vi "TimeDelay.vi"(0 "Ground level BP-filter width, Hz":dbl format="%#_13g", 2 "Generator frequency":dbl format="%#_13g", 3 "Sampling frequency":dbl format="%#_13g") -> (1 "dt":dbl format="%#_13g")   [LabVIEW 2015]
uses:
  <vilib>/measure/maspectr.llb/FFT Spectrum (Mag-Phase) for 1 Chan.vi
  <vilib>/Analysis/3filter.llb/Butterworth Filter (DBL).vi
  <vilib>/measure/NI_MABase.lvlib
  <vilib>/measure/NI_MAPro.lvlib
  <vilib>/Analysis/NI_AALBase.lvlib
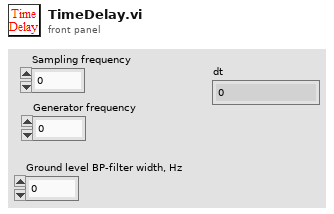
[diagram p1: front panel]
types:
  T1 = cluster{"Sampling frequency":dbl, "Number of samples":dbl}
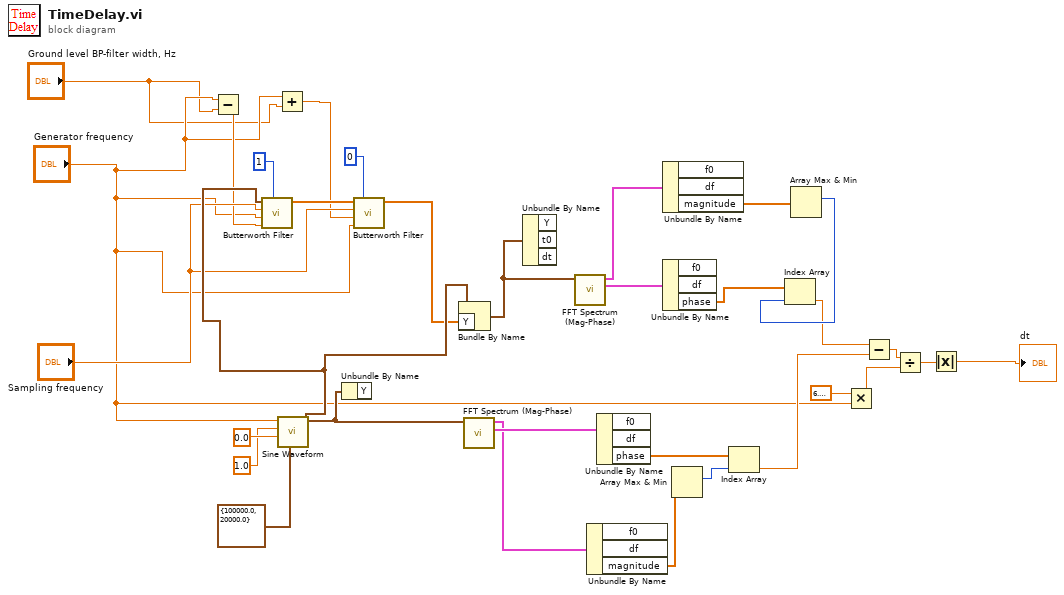
[diagram p0: block diagram]
diagram:
  n1 = Subtract(x="Generator frequency", y="Ground level BP-filter width, Hz") -> (x-y=w5:dbl)
  n2 = Add(x="Generator frequency", y="Ground level BP-filter width, Hz") -> (x+y=w2:dbl)
  n3 = call <vilib>:"Sine Waveform.vi"("sampling info"=T1 {"Sampling frequency"=100000.0, "Number of samples"=20000.0} ("Cluster 2"), "phase"=0.0, "amplitude"=1.0, "frequency"="Generator frequency") -> ("signal out"=w8:waveform(dbl))  [unwired: 6 in, 1 out]
  n4 = call-poly <vilib>:"Butterworth Filter.vi"("filter type"=1, "low cutoff freq: fl"=w5, "high cutoff freq: fh"="Generator frequency", "sampling freq: fs"="Sampling frequency", "X"=w8) -> ("Filtered X"=w11:dbl[])  [unwired: 3 in, 1 out]
  n5 = Unbundle By Name(w8) -> ()  [unwired: 1 out]
  n6 = call-poly <vilib>:"Butterworth Filter.vi"("filter type"=0, "low cutoff freq: fl"="Generator frequency", "high cutoff freq: fh"=w2, "sampling freq: fs"="Sampling frequency", "X"=w11) -> ("Filtered X"=w7:dbl[])  [unwired: 3 in, 1 out]
  n7 = Bundle By Name(cluster=w8, "Y"=w7) -> (w13:waveform(dbl))
  n8 = call-poly <vilib>:"FFT Spectrum (Mag-Phase).vi"("time signal"=w8) -> ("phase"=w30:cluster{"f0":dbl, "df":dbl, "phase":dbl[]}, "magnitude"=w21:cluster{"f0":dbl, "df":dbl, "magnitude":dbl[]})  [unwired: 6 in, 3 out]
  n9 = Unbundle By Name(w13) -> ()  [unwired: 3 out]
  n10 = call-poly <vilib>:"FFT Spectrum (Mag-Phase).vi"("time signal"=w13) -> ("phase"=w29:cluster{"f0":dbl, "df":dbl, "phase":dbl[]}, "magnitude"=w19:cluster{"f0":dbl, "df":dbl, "magnitude":dbl[]})  [unwired: 6 in, 3 out]
  n11 = Unbundle By Name(w21) -> ("magnitude"=w15:dbl[])  [unwired: 2 out]
  n12 = Unbundle By Name(w30) -> ("phase"=w22:dbl[])  [unwired: 2 out]
  n13 = Unbundle By Name(w19) -> ("magnitude"=w16:dbl[])  [unwired: 2 out]
  n14 = Unbundle By Name(w29) -> ("phase"=w18:dbl[])  [unwired: 2 out]
  n15 = Array Max & Min(array=w15) -> (max index (indices)=w20:i32)  [unwired: 3 out]
  n16 = Index Array(array=w22, index=w20) -> (element=w23:dbl)
  n17 = Array Max & Min(array=w16) -> (max index (indices)=w17:i32)  [unwired: 3 out]
  n18 = Index Array(array=w18, index=w17) -> (element=w12:dbl)
  n19 = Multiply(x=6.283185307179586, y="Generator frequency") -> (x*y=w26:dbl)
  n20 = Subtract(x=w12, y=w23) -> (x-y=w28:dbl)
  n21 = Divide(x=w28, y=w26) -> (x/y=w25:dbl)
  n22 = Absolute Value(x=w25) -> (abs(x)=→"dt":dbl)
